vi "采集数据.vi"(8 "error in (no error)":errorcluster caption="错误输入（无错误）", 11 "数据采集 输入":refnum<class "数据采集.lvclass"> caption="DNL_LabVIEW Object in") -> (0 "error out":errorcluster caption="错误输出", 3 "数据采集 输出":refnum<class "数据采集.lvclass"> caption="DNL_LabVIEW Object out")   [LabVIEW 2013, in "数据采集.lvclass"]
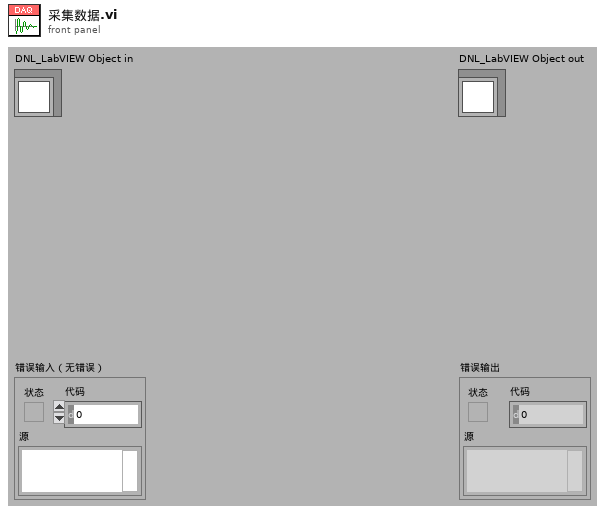
[diagram p1: front panel]
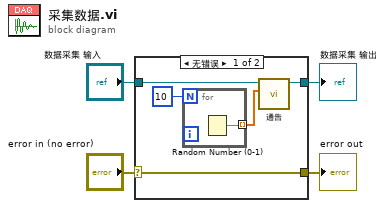
[diagram p0: block diagram]
diagram:
  n1 = case shown="无错误" "error in (no error)" {
    selector: "error in (no error)" -> [w9 w12]
    tunnel: [w9 w12] -> w3
    tunnel: [w5 w11] -> w1
    tunnel: "数据采集 输入" -> [w7 w11]
    frame No Error {
      n2 = for {
        N: 10 -> [_]
        tunnel: [w10] -> w6 mode=indexing
        n3 = Random Number (0-1)() -> (number: 0 to 1=w10:dbl)
      }
      n4 = call-dynamic "通告.vi"("采集数据"=w6, "数据采集 输入"=w7) -> ("数据采集 输出"=w5:refnum<class "数据采集.lvclass">)  [unwired: 8 in, 1 out]
    }
    frame Error {
    }
  }
  "error out" <- w3
  "数据采集 输出" <- w1
